vi "CloseDevice.vi"(1 "Handle":u32) -> (0 "Result":u32)   [LabVIEW 2010]
uses:
  FTCSPI.dll
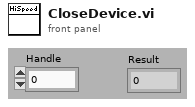
[diagram p1: front panel]
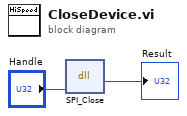
[diagram p0: block diagram]
diagram:
  n1 = dll-call lib="C:/Users/Administrator/Documents/GitHub/labview/FPGA/FTCSPI.dll" fn="SPI_Close"("Handle"="Handle") -> ("FTC_Status"=→"Result":u32)  [unwired: 4 in, 2 out]
